vi "test_XMLlvParser.vi"() -> ()   [LabVIEW 2020]
uses:
  Import/_typedefs/session_rx_monitor.ctl
  Shared/hardware_channels_rx.ctl
  Shared/channel_settings_rx.ctl
  <instrlib>/AIM GmbH/_AIM 664/_controls/session_monitor_config.ctl
  Shared/monitor_queue_settings.ctl
  Shared/loggingThreshold_types.ctl
  Shared/hardware_channels_tx.ctl
  Shared/channel_settings_tx.ctl
  Shared/Frame Payload Parameters.ctl
  Shared/Encoding (Arinc664).ctl
  Shared/RawFrame_entry.ctl
  <instrlib>/AIM GmbH/_AIM 664/_controls/queue_header_generic.ctl
  <instrlib>/AIM GmbH/_AIM 664/AIM664LV.lvlib
  Import/AIM ARINC 664 Import.lvlib
panel:
  out "value":T1 {"channel settings"."Payload Parameter Array"."Parameters"."encoding" items=["BNR", "BCD", "Discrete"]}
  out "error out 2":errorcluster caption="error out"
  out "Tx Generic Configuration":T1 {"channel settings"."Payload Parameter Array"."Parameters"."encoding" items=["BNR", "BCD", "Discrete"]}
  in  "get  tx gen - xml in":string
  out "error out":errorcluster
  out "Rx Mon Configuration":T7={"channel #"=0, "channel handle"=0, "InstrumentHandle_board"=0, "InstrumentHandle_port"=0, "Queue ID"=0, "channel settings"={"Monitor Settings"={"DefaultCronoMode"=0, "GlbMonBufferSizeIn"=0}, "Rx Board"=0, "Rx Port"=0}, "current log file name"=path "", "monitor queue settings"={"TriggerPosition"=0, "CaptureMode"=0, "Strobe"=0, "MaxFileSize MB (1)"=1}, "Log File Directory"="", "Base name"="", "Timestamp"=FALSE, "log thresholds"={"Segmentation Threshold"=0.0, "Disk Space Percentage"=0.0, "Check Disk Space"=FALSE, "Segment File"=FALSE, "Segment Files By"=0}} {"log thresholds"."Segment Files By" items=["Time", "Size"]; "monitor queue settings"."Strobe" items=["FDX_MON_STROBE_DIS", "FDX_MON_STROBE_STOP", "FDX_MON_STROBE_START"]; "monitor queue settings"."CaptureMode" items=["FDX_MON_SINGLE ", "FDX_MON_CONTINUOUS", "FDX_MON_SELECTIVE", "FDX_MON_RECORDING", "FDX_MON_REROS", "FDX_MON_HMU"]; "channel settings"."Monitor Settings"."DefaultCronoMode" items=["FDX_RX_DEFAULT_ENA_CNT", "FDX_RX_DEFAULT_MON_ENA_ALL", "FDX_RX_DEFAULT_MON_ENA_GOOD"]}
  in  "get  mon - xml in":string
  out "error out":errorcluster
  in  "set  tx gen - xml in":string
  out "set xml out":T12={"DefaultCronoMode"=1, "GlbMonBufferSizeIn"=0, "CaptureMode"=0, "MaxFileSizeMB"=1, "Strobe"=0, "TriggerPosition"=0} {"Strobe" items=["FDX_MON_STROBE_DIS", "FDX_MON_STROBE_STOP", "FDX_MON_STROBE_START"]; "CaptureMode" items=["FDX_MON_SINGLE ", "FDX_MON_CONTINUOUS", "FDX_MON_SELECTIVE", "FDX_MON_RECORDING", "FDX_MON_REROS", "FDX_MON_HMU"]; "DefaultCronoMode" items=["FDX_RX_DEFAULT_ENA_CNT", "FDX_RX_DEFAULT_MON_ENA_ALL", "FDX_RX_DEFAULT_MON_ENA_GOOD"]}
  out "error out":errorcluster
  in  "set  mon - xml in":string
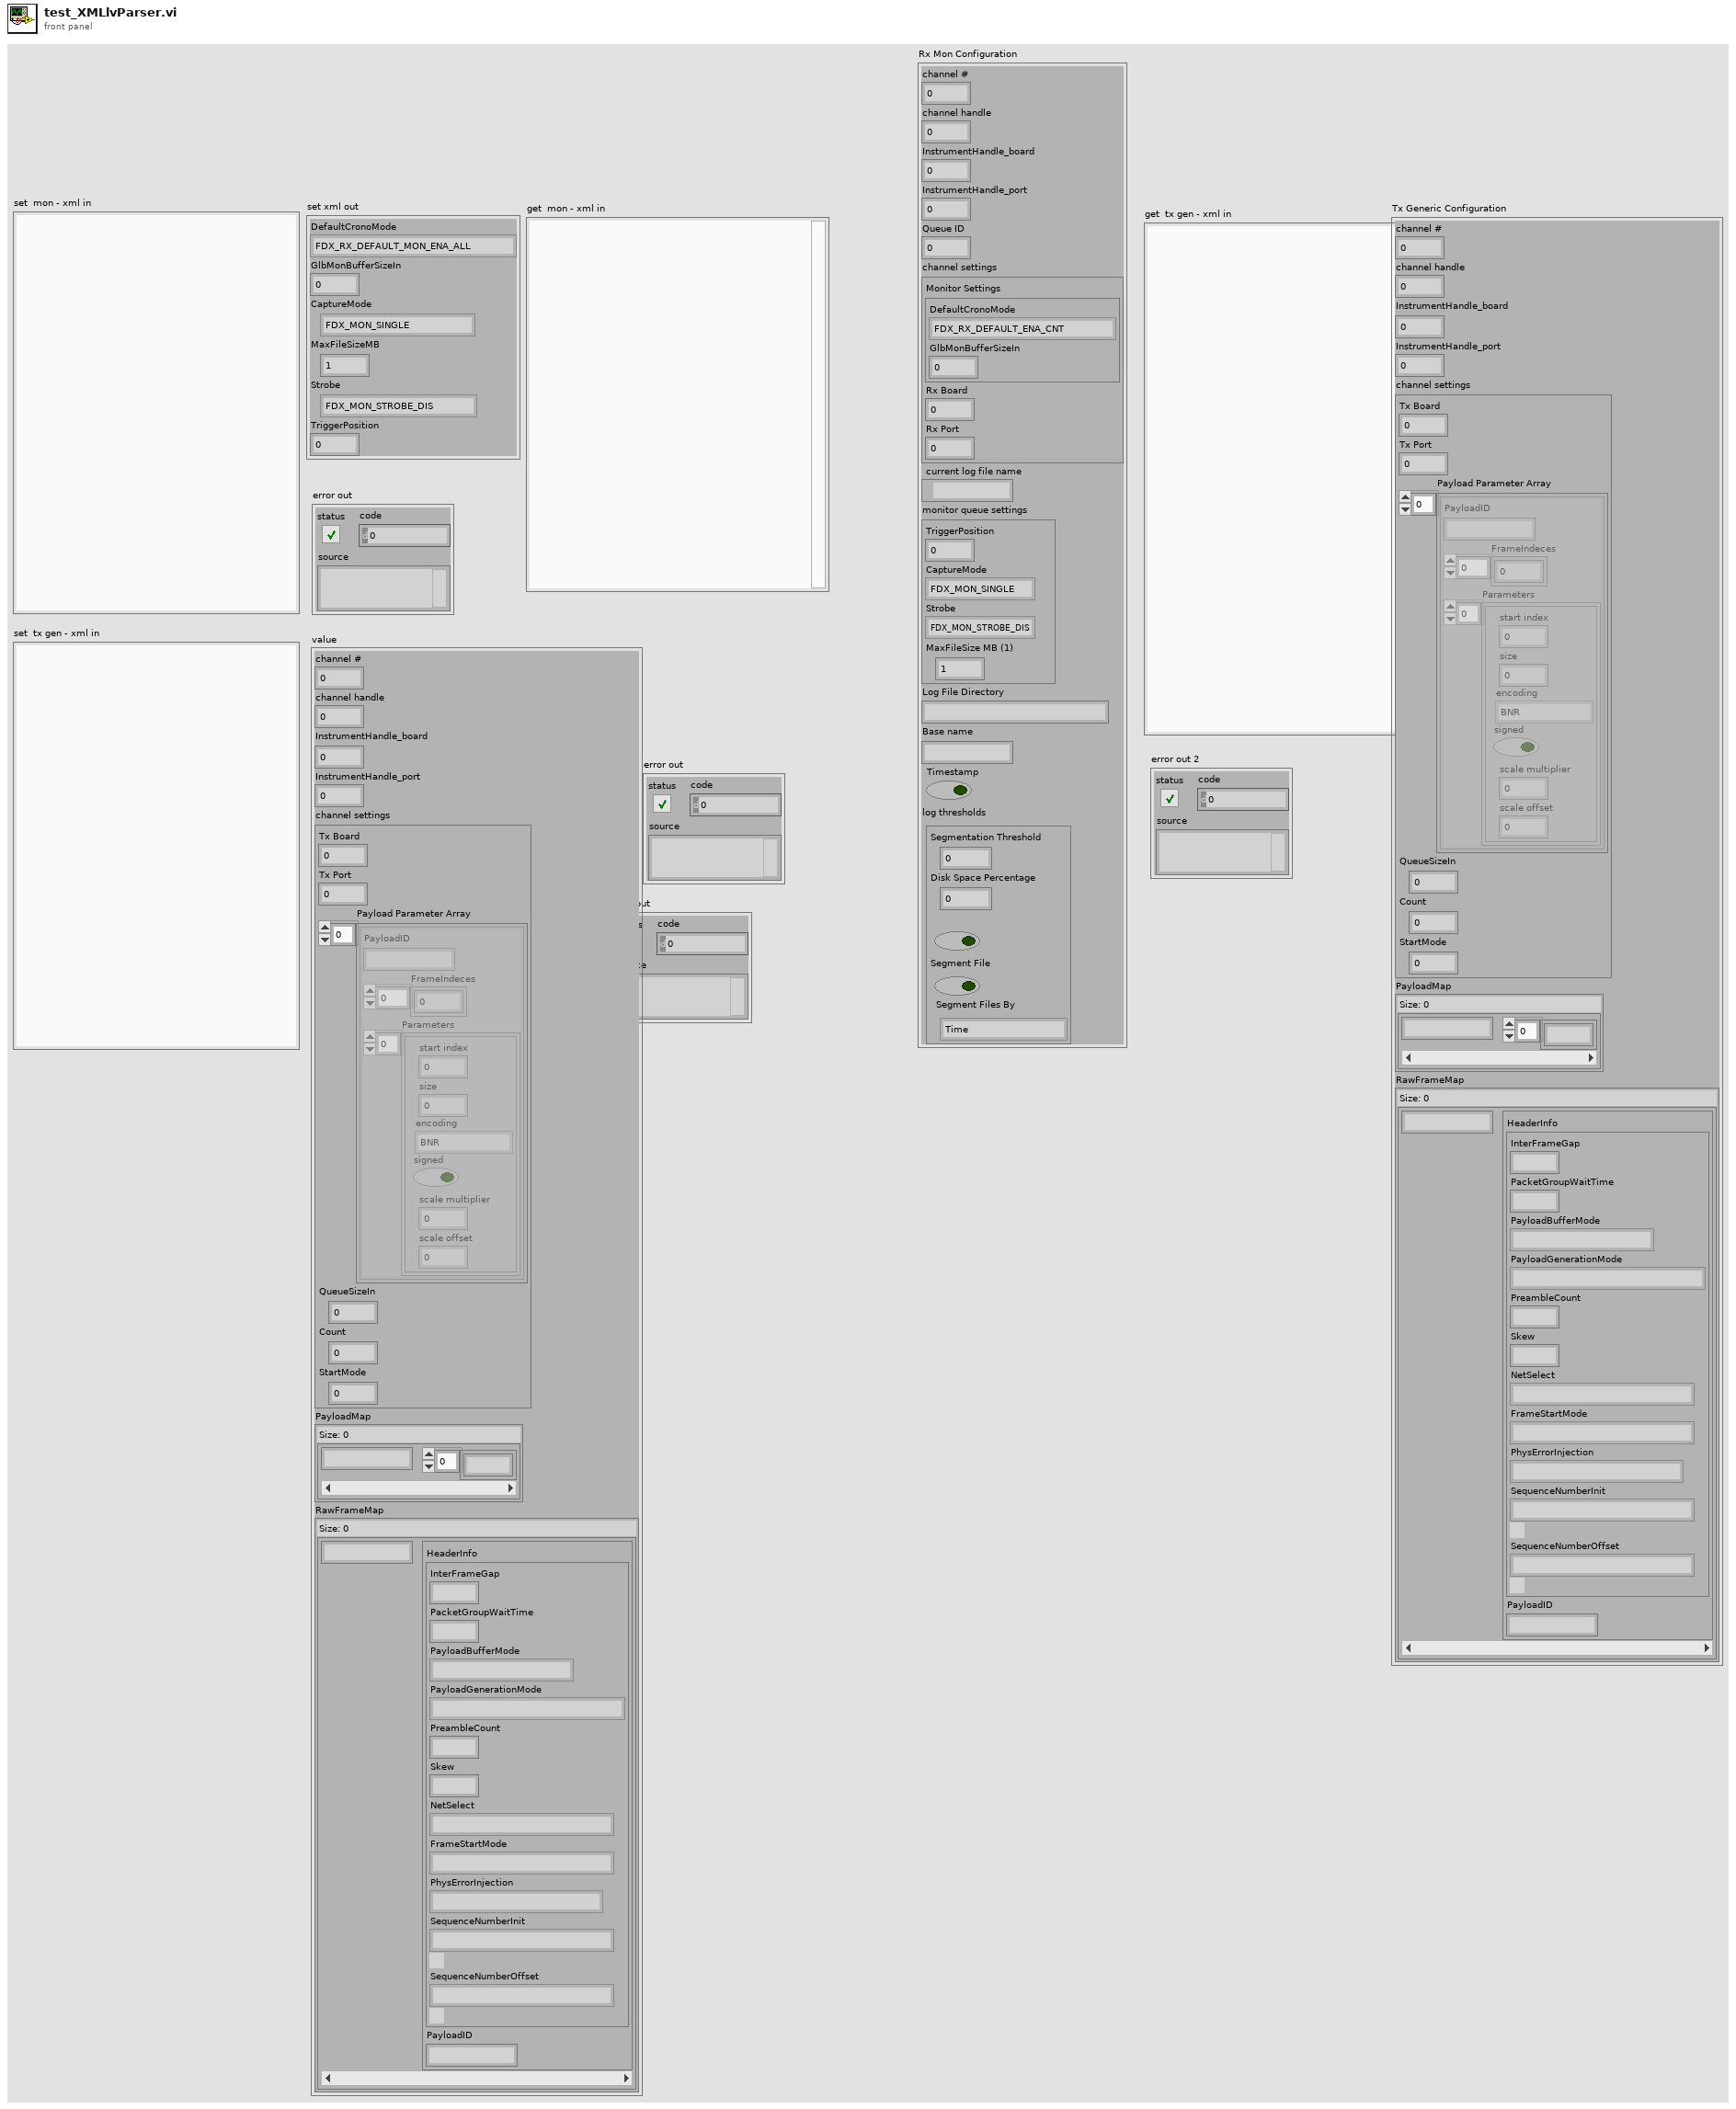
[diagram p1: front panel]
types:
  T1 = typedef "hardware_channels_tx.ctl" = cluster{"channel #":u16, "channel handle":u64, "InstrumentHandle_board":u32, "InstrumentHandle_port":u32, "channel settings":T2, "PayloadMap":map{string, u8[]}, "RawFrameMap":map{string, T5}}
  T2 = typedef "channel_settings_tx.ctl" = cluster{"Tx Board":u32, "Tx Port":u32, "Payload Parameter Array":T3[], "QueueSizeIn":u32, "Count":u32, "StartMode":u32}
  T3 = typedef "Frame Payload Parameters.ctl" = cluster{"PayloadID":string, "FrameIndeces":u32[], "Parameters":cluster{"start index":i32, "size":i32, "encoding":T4, "signed":bool, "scale multiplier":dbl, "scale offset":dbl}[]}
  T4 = typedef "Encoding (Arinc664).ctl" = u16
  T5 = typedef "RawFrame_entry.ctl" = cluster{"HeaderInfo":T6, "PayloadID":string}
  T6 = typedef "AIM664LV.lvlib/queue_header_generic.ctl" = cluster{"InterFrameGap":u32, "PacketGroupWaitTime":u32, "PayloadBufferMode":u8, "PayloadGenerationMode":u8, "PreambleCount":u8, "Skew":u32, "NetSelect":u8, "FrameStartMode":u8, "PhysErrorInjection":u32, "SequenceNumberInit":u16, "SequenceNumberOffset":u16}
  T7 = typedef "hardware_channels_rx.ctl" = cluster{"channel #":u16, "channel handle":u64, "InstrumentHandle_board":u32, "InstrumentHandle_port":u32, "Queue ID":u32, "channel settings":T8, "current log file name":path, "monitor queue settings":T10, "Log File Directory":string, "Base name":string, "Timestamp":bool, "log thresholds":T11}
  T8 = typedef "channel_settings_rx.ctl" = cluster{"Monitor Settings":T9, "Rx Board":u32, "Rx Port":u32}
  T9 = typedef "AIM664LV.lvlib/session_monitor_config.ctl" = cluster{"DefaultCronoMode":u32, "GlbMonBufferSizeIn":u32}
  T10 = typedef "monitor_queue_settings.ctl" = cluster{"TriggerPosition":u32, "CaptureMode":u32, "Strobe":u32, "MaxFileSize MB (1)":u32}
  T11 = typedef "loggingThreshold_types.ctl" = cluster{"Segmentation Threshold":dbl, "Disk Space Percentage":dbl, "Check Disk Space":bool, "Segment File":bool, "Segment Files By":u16}
  T12 = typedef "AIM ARINC 664 Import.lvlib/session_rx_monitor.ctl" = cluster{"DefaultCronoMode":u32, "GlbMonBufferSizeIn":u32, "CaptureMode":u32, "MaxFileSizeMB":u32, "Strobe":u32, "TriggerPosition":u32}
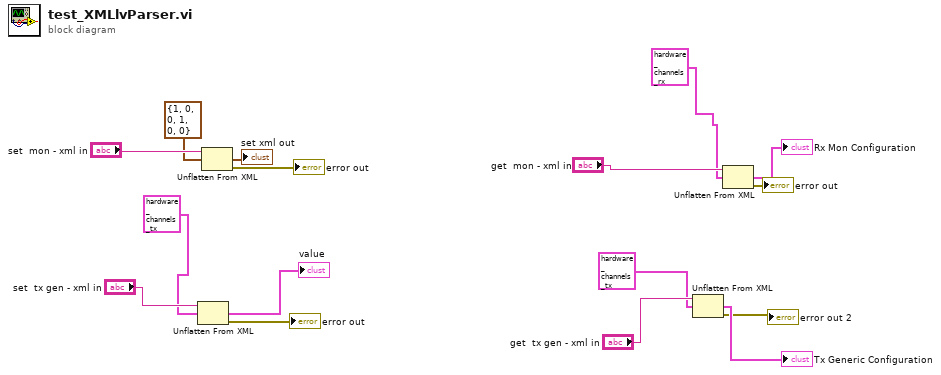
[diagram p0: block diagram]
diagram:
  n1 = Unflatten From XML(xml string="set  tx gen - xml in", type=T1 {"channel #"=0, "channel handle"=0, "InstrumentHandle_board"=0, "InstrumentHandle_port"=0, "channel settings"={"Tx Board"=0, "Tx Port"=0, "Payload Parameter Array"=[], "QueueSizeIn"=0, "Count"=0, "StartMode"=0}, "PayloadMap"={}, "RawFrameMap"={}} ("Tx cluster out")) -> (value=→"value":T1, error out=→"error out":errorcluster)  [unwired: 1 in]
  n2 = Unflatten From XML(xml string="set  mon - xml in", type=T12 {"DefaultCronoMode"=1, "GlbMonBufferSizeIn"=0, "CaptureMode"=0, "MaxFileSizeMB"=1, "Strobe"=0, "TriggerPosition"=0} ("session_rx_monitor")) -> (value=→"set xml out":T12, error out=→"error out":errorcluster)  [unwired: 1 in]
  n3 = Unflatten From XML(xml string="get  tx gen - xml in", type=T1 {"channel #"=0, "channel handle"=0, "InstrumentHandle_board"=0, "InstrumentHandle_port"=0, "channel settings"={"Tx Board"=0, "Tx Port"=0, "Payload Parameter Array"=[], "QueueSizeIn"=0, "Count"=0, "StartMode"=0}, "PayloadMap"={}, "RawFrameMap"={}} ("Tx cluster out")) -> (value=→"Tx Generic Configuration":T1, error out=→"error out 2":errorcluster)  [unwired: 1 in]
  n4 = Unflatten From XML(xml string="get  mon - xml in", type=T7 {"channel #"=0, "channel handle"=0, "InstrumentHandle_board"=0, "InstrumentHandle_port"=0, "Queue ID"=0, "channel settings"={"Monitor Settings"={"DefaultCronoMode"=0, "GlbMonBufferSizeIn"=0}, "Rx Board"=0, "Rx Port"=0}, "current log file name"=path "", "monitor queue settings"={"TriggerPosition"=0, "CaptureMode"=0, "Strobe"=0, "MaxFileSize MB (1)"=1}, "Log File Directory"="", "Base name"="", "Timestamp"=FALSE, "log thresholds"={"Segmentation Threshold"=0.0, "Disk Space Percentage"=0.0, "Check Disk Space"=FALSE, "Segment File"=FALSE, "Segment Files By"=0}} ("Monitor cluster out")) -> (value=→"Rx Mon Configuration":T7, error out=→"error out":errorcluster)  [unwired: 1 in]
